vi "Zr_control_to_VCH.vi"(10 "Z_ASetState":T1, 11 "Zr_control":T3) -> (2 "Reset_ALR":bool, 3 "Z_control":T2)   [LabVIEW 2019, in "Valves.lvlib"]
uses:
  Valves.lvlib
  ctl/Z_State_VCH.ctl
  ctl/Z_control_VCH.ctl
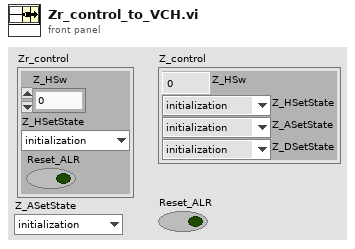
[diagram p1: front panel]
types:
  T1 = typedef "Valves.lvlib/Z_State_VCH.ctl" = enum8{"initialization", "alarm", "disabled", "not ready", "closed ready", "reserv", "reserv1", "reserv2", "reserv3", "check", "on min", "open", "on (closed)"}
  T2 = typedef "Valves.lvlib/Z_control_VCH.ctl" = cluster{"Z_HSw":u8, "Z_HSetState":T1, "Z_ASetState":T1, "Z_DSetState":T1}
  T3 = cluster{"Z_HSw":u8, "Z_HSetState":T1, "Reset_ALR":bool}
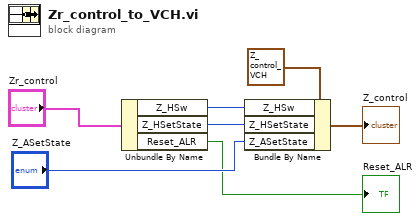
[diagram p0: block diagram]
diagram:
  n1 = Unbundle By Name("Zr_control") -> ("Z_HSw"=w4:u8, "Z_HSetState"=w3:T1, "Reset_ALR"=→"Reset_ALR":bool)
  n2 = Bundle By Name(cluster=T2 {"Z_HSw"=1, "Z_HSetState"=enum."on (closed)", "Z_ASetState"=enum."on (closed)", "Z_DSetState"=enum."on (closed)"} ("Z_control"), "Z_HSw"=w4, "Z_HSetState"=w3, "Z_ASetState"="Z_ASetState") -> (→"Z_control":T2)
